vi "Calculate Vertex Array.vi"(8 "error in (no error)":errorcluster, 9 "Coordinates System":enum16{"Cartesian", "Cylindrical", "Spherical"}(ring)=enum."Spherical", 10 "3D Stem Datatype.lvclass in":refnum<class "3D Stem Datatype.lvclass">, 11 "Plot Representation In":T1) -> (0 "error out":errorcluster, 1 "Dup Coordinates System":enum16{"Cartesian", "Cylindrical", "Spherical"}(ring)=enum."Spherical", 2 "3D Stem Datatype.lvclass out":refnum<class "3D Stem Datatype.lvclass">, 3 "Plot Representation Out":T1)   [LabVIEW 2017, in "3D Stem Datatype.lvclass"]
uses:
  <vilib>/Math Plots/3D Math Plots/3D Stem/3D Stem Datatype/3D Stem Datatype.lvclass
  <vilib>/Math Plots/3D Math Plots/3D Plot/3D Plot/Typedef/Plot Representation.ctl
  <vilib>/Math Plots/3D Math Plots/3D Plot/3D Plot/Typedef/Range Clusters.ctl
  <vilib>/Math Plots/3D Math Plots/3D Plot/3D Plot/Typedef/Mesh Data.ctl
  <vilib>/Math Plots/3D Math Plots/3D Stem/3D Stem Datatype/3D Stem Datatype.lvclass/3D Stem Datatype.ctl
  <vilib>/Math Plots/3D Math Plots/3D Plot/3D Plot Datatype/3D Plot Datatype.lvclass
  <vilib>/Math Plots/3D Math Plots/3D Plot/3D Plot/3D Plot.lvclass
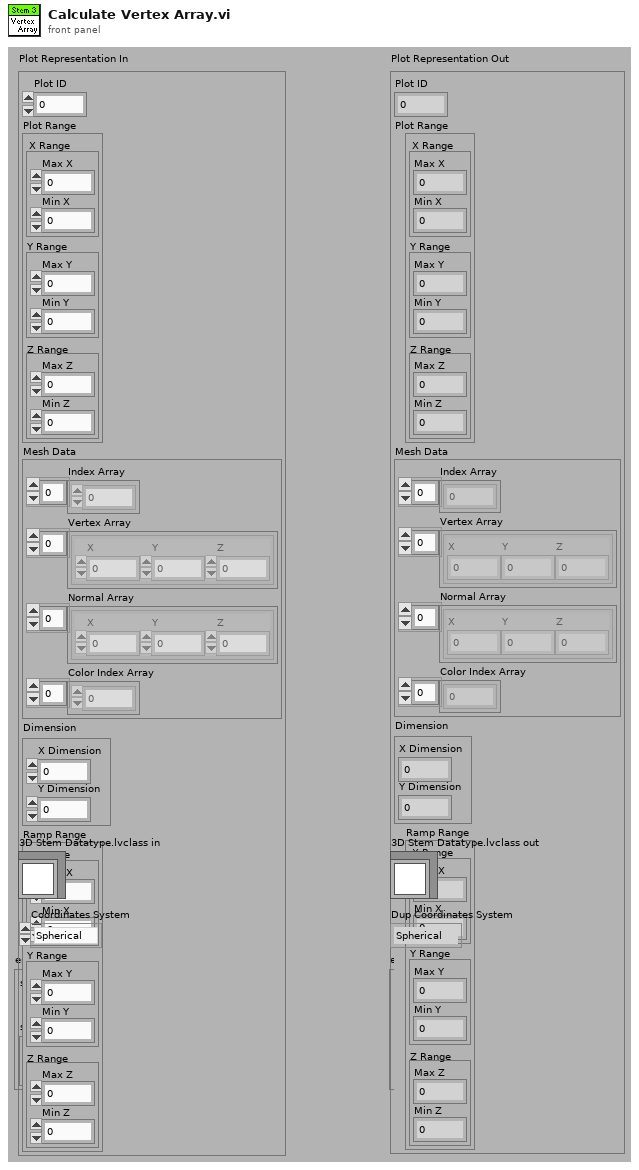
[diagram p1: front panel]
types:
  T1 = typedef "3D Plot.lvclass/Plot Representation.ctl" = cluster{"Plot ID":i32, "Plot Range":T2, "Mesh Data":T3, "Dimension":cluster{"X Dimension":i32, "Y Dimension":i32}, "Ramp Range":T2}
  T2 = typedef "3D Plot.lvclass/Range Clusters.ctl" = cluster{"X Range":cluster{"Max X":sgl, "Min X":sgl}, "Y Range":cluster{"Max Y":sgl, "Min Y":sgl}, "Z Range":cluster{"Max Z":sgl, "Min Z":sgl}}
  T3 = typedef "3D Plot.lvclass/Mesh Data.ctl" = cluster{"Index Array":u32[], "Vertex Array":cluster{"X":sgl, "Y":sgl, "Z":sgl}[], "Normal Array":cluster{"X":sgl, "Y":sgl, "Z":sgl}[], "Color Index Array":i32[]}
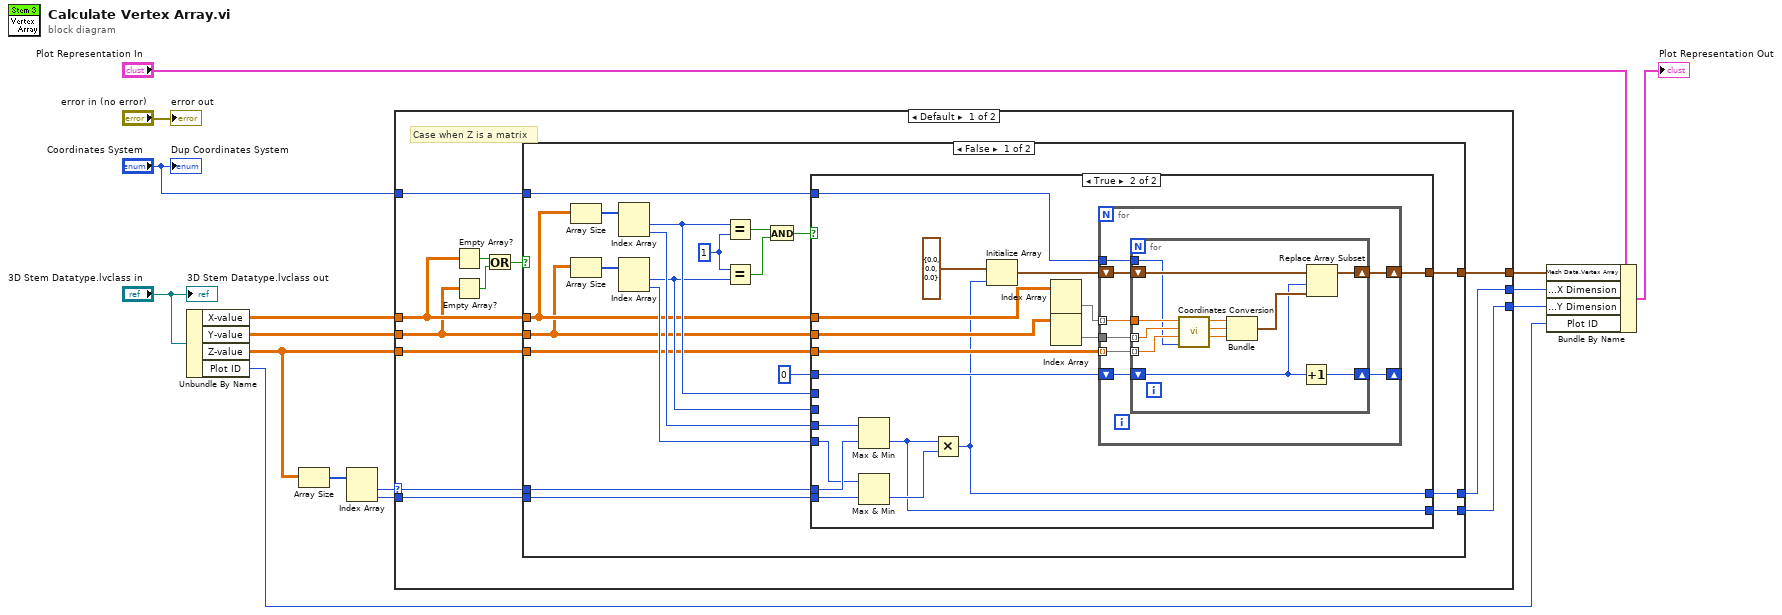
[diagram p0: block diagram]
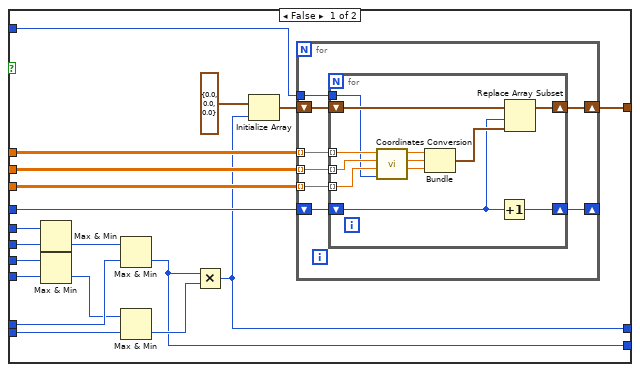
[diagram p2: hidden frame]
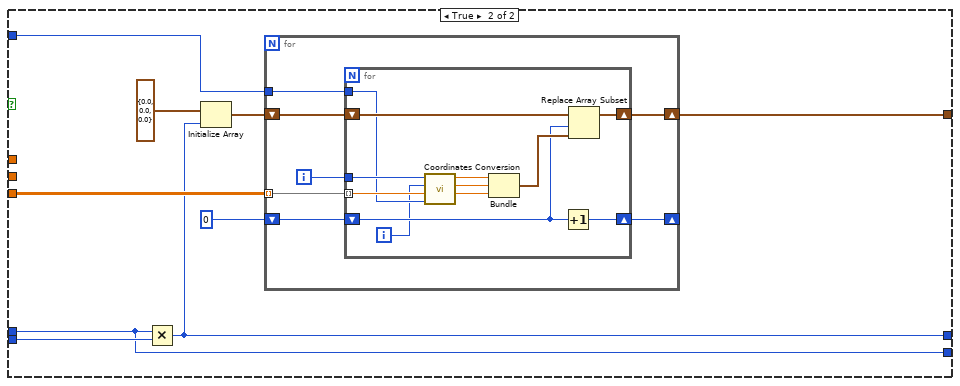
[diagram p3: hidden frame]
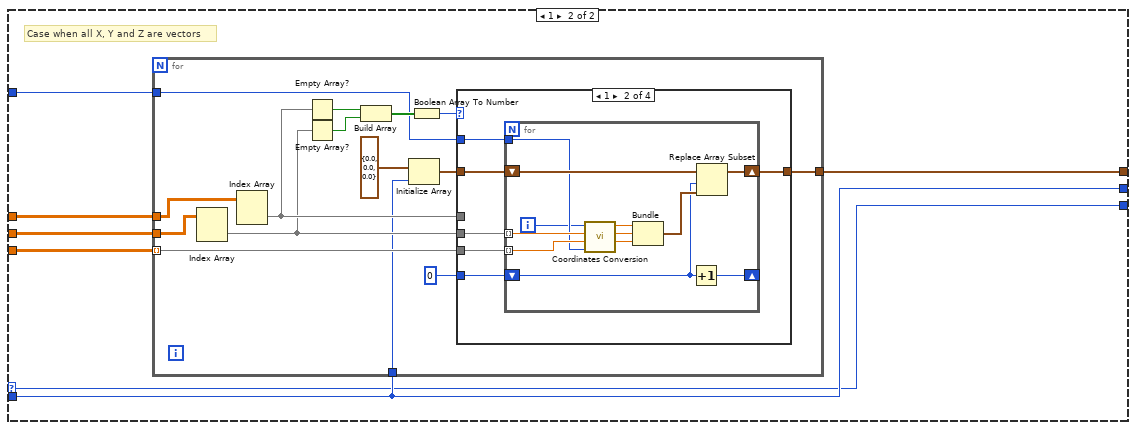
[diagram p4: hidden frame]
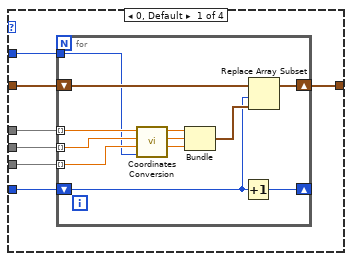
[diagram p5: hidden frame]
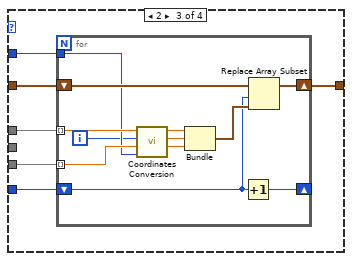
[diagram p6: hidden frame]
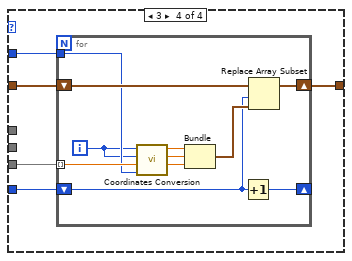
[diagram p7: hidden frame]
diagram:
  n1 = Unbundle By Name("3D Stem Datatype.lvclass in") -> ("X-value"=w9:sgl[][], "Y-value"=w10:sgl[][], "Z-value"=w11:sgl[][], "Plot ID"=w6:i32)
  n2 = Array Size(array=w11) -> (size(s)=w7:i32[])
  n3 = Index Array(array=w7) -> (element #1=w8:i32, element #2=w12:i32)  [unwired: 2 in]
  n4 = case shown="Default" w8 {
    selector: w8 -> [w20 w152]
    tunnel: w9 -> [w23 w158]
    tunnel: w10 -> [w22 w157]
    tunnel: w11 -> [w21 w156]
    tunnel: "Coordinates System" -> [w27 w155]
    tunnel: w12 -> [w19 w153]
    tunnel: [w18 w153] -> w13
    tunnel: [w17 w154] -> w14
    tunnel: [w16 w152] -> w1
    frame Default {
      # "Case when Z is a matrix"
      n5 = Empty Array?(array=w23) -> (empty?=w25:bool)
      n6 = Empty Array?(array=w22) -> (empty?=w26:bool)
      n7 = Or(x=w25, y=w26) -> (x .or. y?=w24:bool)
      n8 = case shown="False" w24 {
        tunnel: [w30 w132] -> w17
        tunnel: w20 -> [w32 w124]
        tunnel: w21 -> [w33 w131]
        tunnel: w27 -> [w36 w130]
        tunnel: [w29 w125] -> w18
        tunnel: w23 -> [w35 _]
        tunnel: w22 -> [w34 _]
        tunnel: w19 -> [w31 w126]
        tunnel: [w28 w124] -> w16
        frame False {
          w45 = 1 ("x")
          n9 = Array Size(array=w35) -> (size(s)=w47:i32[])
          n10 = Array Size(array=w34) -> (size(s)=w46:i32[])
          n11 = Index Array(array=w47) -> (element #1=w38:i32, element #2=w40:i32)  [unwired: 2 in]
          n12 = Index Array(array=w46) -> (element #1=w37:i32, element #2=w39:i32)  [unwired: 2 in]
          n13 = Equal?(x=w38, y=w45) -> (x = y?=w44:bool)
          n14 = Equal?(x=w45, y=w37) -> (x = y?=w43:bool)
          n15 = And(x=w44, y=w43) -> (x .and. y?=w42:bool)
          n16 = case shown="True" w42 {
            tunnel: w36 -> [w66 w103]
            tunnel: w35 -> [w65 w99]
            tunnel: w34 -> [w64 w98]
            tunnel: w33 -> [w63 w100]
            tunnel: 0 -> [w62 w101]
            tunnel: [w61 w102] -> w30
            tunnel: w40 -> [w56 w93]
            tunnel: w32 -> [w53 w92]
            tunnel: w39 -> [w55 w91]
            tunnel: w31 -> [w51 w90]
            tunnel: [w49 w88] -> w29
            tunnel: w38 -> [w58 _]
            tunnel: w37 -> [w57 _]
            tunnel: [w48 w87] -> w28
            frame False {
              n17 = Max & Min(x=w58, y=w57) -> (min(x,y)=w54:i32)  [unwired: 1 out]
              n18 = Max & Min(x=w56, y=w55) -> (min(x,y)=w52:i32)  [unwired: 1 out]
              n19 = Max & Min(x=w54, y=w53) -> (min(x,y)=w48:i32)  [unwired: 1 out]
              n20 = Max & Min(x=w52, y=w51) -> (min(x,y)=w50:i32)  [unwired: 1 out]
              n21 = Multiply(x=w48, y=w50) -> (x*y=w49:i32)
              n22 = Initialize Array(cluster{"X":sgl, "Y":sgl, "Z":sgl} {"X"=0.0, "Y"=0.0, "Z"=0.0} ("3D Point"), w49) -> (w59:cluster{"X":sgl, "Y":sgl, "Z":sgl}[])
              n23 = for {
                shift-right: [w73] -> w61
                shift-left: w59 -> [w74]
                tunnel: w63 -> [w72] mode=indexing
                tunnel: w65 -> [w70] mode=indexing
                tunnel: w64 -> [w71] mode=indexing
                tunnel: w66 -> [w69]
                shift-right: [w67] -> _
                shift-left: w62 -> [w68]
                n24 = for {
                  tunnel: w72 -> [w82] mode=indexing
                  shift-right: [w86] -> w73
                  shift-left: w74 -> [w85]
                  tunnel: w71 -> [w83] mode=indexing
                  tunnel: w70 -> [w84] mode=indexing
                  tunnel: w69 -> [w78]
                  shift-right: [w76] -> w67
                  shift-left: w68 -> [w75]
                  n25 = call <vilib>:"Coordinates Conversion.vi"("Coordinates System"=w78, "Z in"=w82, "Y in"=w83, "X in"=w84) -> ("Z out"=w79:sgl, "Y out"=w80:sgl, "X out"=w81:sgl)  [unwired: 5 out]
                  n26 = Bundle("X out"=w81, "Y out"=w80, "Z out"=w79) -> (w77:cluster{"X out":sgl, "Y out":sgl, "Z out":sgl})  [unwired: 1 out]
                  n27 = Increment(x=w75) -> (x+1=w76:i32)
                  n28 = Replace Array Subset(array=w85, new element=w77, index=w75) -> (w86:cluster{"X":sgl, "Y":sgl, "Z":sgl}[])
                }
              }
            }
            frame True {
              n29 = Max & Min(x=w93, y=w92) -> (min(x,y)=w87:i32)  [unwired: 1 out]
              n30 = Max & Min(x=w91, y=w90) -> (min(x,y)=w89:i32)  [unwired: 1 out]
              n31 = Multiply(x=w87, y=w89) -> (x*y=w88:i32)
              n32 = Initialize Array(cluster{"X":sgl, "Y":sgl, "Z":sgl} {"X"=0.0, "Y"=0.0, "Z"=0.0} ("3D Point"), w88) -> (w94:cluster{"X":sgl, "Y":sgl, "Z":sgl}[])
              n33 = Index Array(array=w99) -> (element=w96:sgl[])  [unwired: 2 in]
              n34 = Index Array(array=w98) -> (element=w97:sgl[])  [unwired: 2 in]
              n35 = for {
                shift-right: [w110] -> w102
                shift-left: w94 -> [w111]
                tunnel: w100 -> [w109] mode=indexing
                tunnel: w96 -> [w107] mode=indexing
                tunnel: w97 -> [w108]
                tunnel: w103 -> [w106]
                shift-right: [w104] -> _
                shift-left: w101 -> [w105]
                n36 = for {
                  tunnel: w109 -> [w119] mode=indexing
                  shift-right: [w123] -> w110
                  shift-left: w111 -> [w122]
                  tunnel: w108 -> [w120] mode=indexing
                  tunnel: w107 -> [w121]
                  tunnel: w106 -> [w115]
                  shift-right: [w113] -> w104
                  shift-left: w105 -> [w112]
                  n37 = call <vilib>:"Coordinates Conversion.vi"("Coordinates System"=w115, "Z in"=w119, "Y in"=w120, "X in"=w121) -> ("Z out"=w116:sgl, "Y out"=w117:sgl, "X out"=w118:sgl)  [unwired: 5 out]
                  n38 = Bundle("X out"=w118, "Y out"=w117, "Z out"=w116) -> (w114:cluster{"X out":sgl, "Y out":sgl, "Z out":sgl})  [unwired: 1 out]
                  n39 = Increment(x=w112) -> (x+1=w113:i32)
                  n40 = Replace Array Subset(array=w122, new element=w114, index=w112) -> (w123:cluster{"X":sgl, "Y":sgl, "Z":sgl}[])
                }
              }
            }
          }
        }
        frame True {
          n41 = Multiply(x=w124, y=w126) -> (x*y=w125:i32)
          n42 = Initialize Array(cluster{"X":sgl, "Y":sgl, "Z":sgl} {"X"=0.0, "Y"=0.0, "Z"=0.0} ("3D Point"), w125) -> (w128:cluster{"X":sgl, "Y":sgl, "Z":sgl}[])
          n43 = for {
            shift-right: [w138] -> w132
            shift-left: w128 -> [w139]
            tunnel: w131 -> [w137] mode=indexing
            tunnel: w130 -> [w136]
            shift-right: [w134] -> _
            shift-left: 0 -> [w135]
            i -> [w133]
            n44 = for {
              tunnel: w137 -> [w148] mode=indexing
              shift-right: [w151] -> w138
              shift-left: w139 -> [w150]
              tunnel: w133 -> [w149]
              tunnel: w136 -> [w144]
              shift-right: [w142] -> w134
              shift-left: w135 -> [w141]
              i -> [w140]
              n45 = call <vilib>:"Coordinates Conversion.vi"("Coordinates System"=w144, "Z in"=w148, "Y in"=w140, "X in"=w149) -> ("Z out"=w145:sgl, "Y out"=w146:sgl, "X out"=w147:sgl)  [unwired: 5 out]
              n46 = Bundle("X out"=w147, "Y out"=w146, "Z out"=w145) -> (w143:cluster{"X out":sgl, "Y out":sgl, "Z out":sgl})  [unwired: 1 out]
              n47 = Increment(x=w141) -> (x+1=w142:i32)
              n48 = Replace Array Subset(array=w150, new element=w143, index=w141) -> (w151:cluster{"X":sgl, "Y":sgl, "Z":sgl}[])
            }
          }
        }
      }
    }
    frame 1 {
      # "Case when all X, Y and Z are vectors"
      n49 = for {
        tunnel: w158 -> [w163]
        tunnel: w157 -> [w162]
        tunnel: w156 -> [w166] mode=indexing
        tunnel: w155 -> [w165]
        tunnel: [w164] -> w154
        tunnel: w153 -> [w159]
        n50 = Index Array(array=w162) -> (element=w160:sgl[])  [unwired: 2 in]
        n51 = Index Array(array=w163) -> (element=w161:sgl[])  [unwired: 2 in]
        n52 = Empty Array?(array=w161) -> (empty?=w168:bool)
        n53 = Empty Array?(array=w160) -> (empty?=w169:bool)
        n54 = Build Array(w168, w169) -> (w170:bool[])
        n55 = Initialize Array(cluster{"X":sgl, "Y":sgl, "Z":sgl} {"X"=0.0, "Y"=0.0, "Z"=0.0} ("3D Point"), w159) -> (w172:cluster{"X":sgl, "Y":sgl, "Z":sgl}[])
        n56 = Boolean Array To Number(Boolean array=w170) -> (number=w167:u32)
        n57 = case shown="1" w167 {
          tunnel: [w180 w198 w216 w233] -> w164
          tunnel: w172 -> [w179 w197 w215 w232]
          tunnel: 0 -> [w178 w196 w214 w231]
          tunnel: w166 -> [w177 w195 w213 w230]
          tunnel: w161 -> [w176 _ w212 _]
          tunnel: w160 -> [w175 w194 _ _]
          tunnel: w165 -> [w174 w193 w211 w229]
          frame 0, Default {
            n58 = for {
              shift-right: [w191] -> w180
              shift-left: w179 -> [w192]
              tunnel: w177 -> [w188] mode=indexing
              tunnel: w176 -> [w190] mode=indexing
              tunnel: w175 -> [w189] mode=indexing
              tunnel: w174 -> [w184]
              shift-right: [w182] -> _
              shift-left: w178 -> [w181]
              n59 = call <vilib>:"Coordinates Conversion.vi"("Coordinates System"=w184, "Z in"=w188, "Y in"=w189, "X in"=w190) -> ("Z out"=w185:sgl, "Y out"=w186:sgl, "X out"=w187:sgl)  [unwired: 5 out]
              n60 = Bundle("X out"=w187, "Y out"=w186, "Z out"=w185) -> (w183:cluster{"X out":sgl, "Y out":sgl, "Z out":sgl})  [unwired: 1 out]
              n61 = Increment(x=w181) -> (x+1=w182:i32)
              n62 = Replace Array Subset(array=w192, new element=w183, index=w181) -> (w191:cluster{"X":sgl, "Y":sgl, "Z":sgl}[])
            }
          }
          frame 1 {
            n63 = for {
              shift-right: [w209] -> w198
              shift-left: w197 -> [w210]
              tunnel: w195 -> [w207] mode=indexing
              tunnel: w194 -> [w208] mode=indexing
              tunnel: w193 -> [w203]
              shift-right: [w201] -> _
              shift-left: w196 -> [w200]
              i -> [w199]
              n64 = call <vilib>:"Coordinates Conversion.vi"("Coordinates System"=w203, "Z in"=w207, "Y in"=w208, "X in"=w199) -> ("Z out"=w204:sgl, "Y out"=w205:sgl, "X out"=w206:sgl)  [unwired: 5 out]
              n65 = Bundle("X out"=w206, "Y out"=w205, "Z out"=w204) -> (w202:cluster{"X out":sgl, "Y out":sgl, "Z out":sgl})  [unwired: 1 out]
              n66 = Increment(x=w200) -> (x+1=w201:i32)
              n67 = Replace Array Subset(array=w210, new element=w202, index=w200) -> (w209:cluster{"X":sgl, "Y":sgl, "Z":sgl}[])
            }
          }
          frame 2 {
            n68 = for {
              shift-right: [w227] -> w216
              shift-left: w215 -> [w228]
              tunnel: w213 -> [w225] mode=indexing
              tunnel: w212 -> [w226] mode=indexing
              tunnel: w211 -> [w221]
              shift-right: [w219] -> _
              shift-left: w214 -> [w218]
              i -> [w217]
              n69 = call <vilib>:"Coordinates Conversion.vi"("Coordinates System"=w221, "Z in"=w225, "Y in"=w217, "X in"=w226) -> ("Z out"=w222:sgl, "Y out"=w223:sgl, "X out"=w224:sgl)  [unwired: 5 out]
              n70 = Bundle("X out"=w224, "Y out"=w223, "Z out"=w222) -> (w220:cluster{"X out":sgl, "Y out":sgl, "Z out":sgl})  [unwired: 1 out]
              n71 = Increment(x=w218) -> (x+1=w219:i32)
              n72 = Replace Array Subset(array=w228, new element=w220, index=w218) -> (w227:cluster{"X":sgl, "Y":sgl, "Z":sgl}[])
            }
          }
          frame 3 {
            n73 = for {
              shift-right: [w243] -> w233
              shift-left: w232 -> [w244]
              tunnel: w230 -> [w242] mode=indexing
              tunnel: w229 -> [w238]
              shift-right: [w236] -> _
              shift-left: w231 -> [w235]
              i -> [w234]
              n74 = call <vilib>:"Coordinates Conversion.vi"("Coordinates System"=w238, "Z in"=w242, "Y in"=w234, "X in"=w234) -> ("Z out"=w239:sgl, "Y out"=w240:sgl, "X out"=w241:sgl)  [unwired: 5 out]
              n75 = Bundle("X out"=w241, "Y out"=w240, "Z out"=w239) -> (w237:cluster{"X out":sgl, "Y out":sgl, "Z out":sgl})  [unwired: 1 out]
              n76 = Increment(x=w235) -> (x+1=w236:i32)
              n77 = Replace Array Subset(array=w244, new element=w237, index=w235) -> (w243:cluster{"X":sgl, "Y":sgl, "Z":sgl}[])
            }
          }
        }
      }
    }
  }
  n78 = Bundle By Name(cluster="Plot Representation In", "Mesh Data.Vertex Array"=w14, "Dimension.X Dimension"=w13, "Dimension.Y Dimension"=w1, "Plot ID"=w6) -> (→"Plot Representation Out":T1)
  "error out" <- "error in (no error)"
  "3D Stem Datatype.lvclass out" <- "3D Stem Datatype.lvclass in"
  "Dup Coordinates System" <- "Coordinates System"
